vi "Config - Read.vi"(8 "error in (no error)":errorcluster) -> (0 "error out":errorcluster, 3 "Config Records":T1[](array[typedef]))   [LabVIEW 2017]
doc: "Provide reading operation for configuration database process."
uses:
  Controls/Config Record.ctl
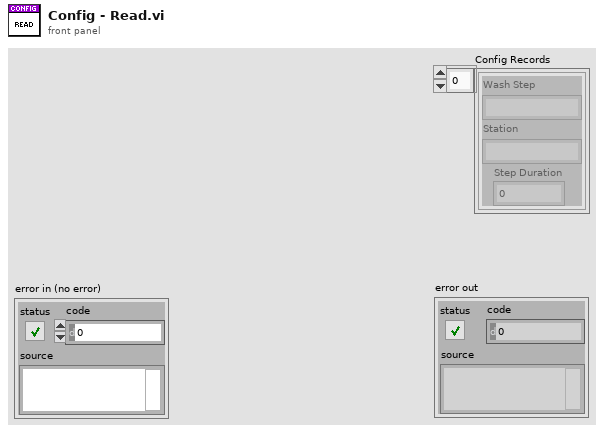
[diagram p1: front panel]
types:
  T1 = typedef "Config Record.ctl" = cluster{"Wash Step":string, "Station":string, "Step Duration":u32}
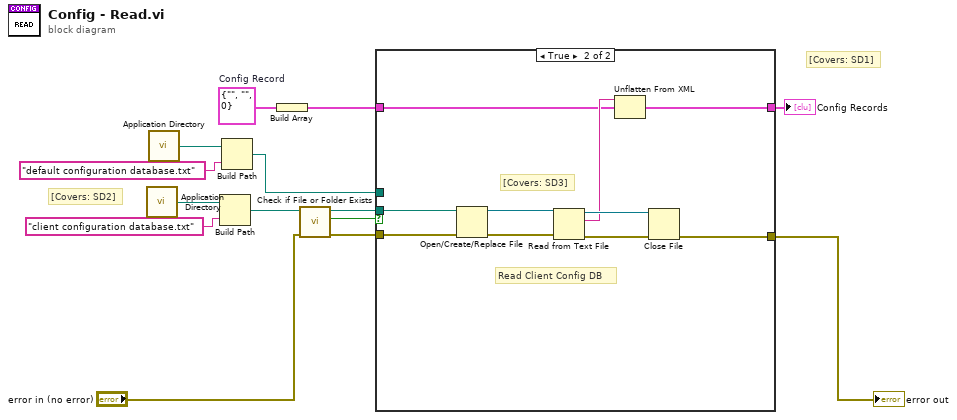
[diagram p0: block diagram]
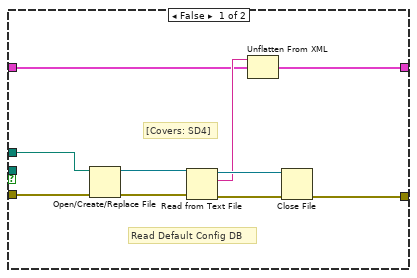
[diagram p2: hidden frame]
diagram:
  w3 = T1 {"Wash Step"="", "Station"="", "Step Duration"=0}  # Config Record
  # "[Covers: SD1]"
  # "[Covers: SD2]"
  n1 = call <vilib>:"Application Directory.vi"() -> ("Application Directory"=w14:path)
  n2 = call <vilib>:"Application Directory.vi"() -> ("Application Directory"=w11:path)
  n3 = Build Path(base path=w14, name or relative path="client configuration database.txt") -> (appended path=w10:path)
  n4 = Build Path(base path=w11, name or relative path="default configuration database.txt") -> (appended path=w5:path)
  n5 = Build Array(w3) -> (w2:T1[])
  n6 = call <vilib>:"Check if File or Folder Exists.vi"("error in (no error)"="error in (no error)", "path"=w10) -> ("error out"=w7:errorcluster, "file or folder exists?"=w9:bool, "dup path"=w8:path)  [unwired: 7 in]
  n7 = case shown="True" w9 {
    tunnel: w8 -> [_ w25]
    tunnel: w7 -> [w24 w34]
    tunnel: w5 -> [w18 _]
    tunnel: [w19 w29] -> w4
    tunnel: [w15 w26] -> w1
    tunnel: w2 -> [w16 w27]
    frame False {
      # "[Covers: SD4]"
      # "Read Default Config DB"
      n8 = Open/Create/Replace File(file path (use dialog)=w18, error in=w24) -> (refnum out=w22:refnum<file>, error out=w23:errorcluster)  [unwired: 4 in, 1 out]
      n9 = Read from Text File(file (use dialog)=w22, error in=w23) -> (refnum out=w20:refnum<file>, text=w17:string, error out=w21:errorcluster)  [unwired: 2 in, 1 out]
      n10 = Unflatten From XML(xml string=w17, type=w16) -> (value=w15:T1[])  [unwired: 1 in, 1 out]
      n11 = Close File(refnum=w20, error in=w21) -> (error out=w19:errorcluster)  [unwired: 1 out]
    }
    frame True {
      # "[Covers: SD3]"
      # "Read Client Config DB"
      n12 = Open/Create/Replace File(file path (use dialog)=w25, error in=w34) -> (refnum out=w32:refnum<file>, error out=w33:errorcluster)  [unwired: 4 in, 1 out]
      n13 = Read from Text File(file (use dialog)=w32, error in=w33) -> (refnum out=w30:refnum<file>, text=w28:string, error out=w31:errorcluster)  [unwired: 2 in, 1 out]
      n14 = Unflatten From XML(xml string=w28, type=w27) -> (value=w26:T1[])  [unwired: 1 in, 1 out]
      n15 = Close File(refnum=w30, error in=w31) -> (error out=w29:errorcluster)  [unwired: 1 out]
    }
  }
  "error out" <- w4
  "Config Records" <- w1
